vi "Run.vi"(7 "Team Index":i32, 8 "Column":i32, 9 "Row":i32, 10 "View":i32[](array[numeric]) caption="View (Team Index, -1: empty)", 11 "Fortress In":refnum<class "Fortress.lvclass">) -> (0 "Replicated":refnum<class "Square.lvclass">, 1 "Direction":T1, 2 "Action":T2, 3 "Square Out":refnum<class "Square.lvclass">)   [LabVIEW 2015, in "Fortress.lvclass"]
uses:
  Fortress.lvclass
  Square/Square.lvclass
  Type Defs/Action Enum.ctl
  Type Defs/Direction Enum.ctl
  Starter/Starter.lvclass
  Fortress.lvclass/Fortress.ctl
  Common/Common.lvlib
  Type Defs/SB Type Defs.lvlib
panel:
  # "NW\nN\nNE\nE\nSE\nS\nSW\nW"
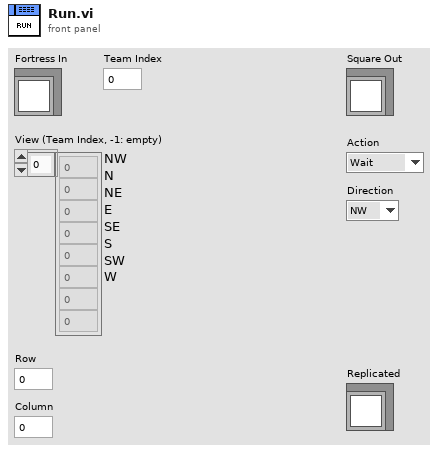
[diagram p1: front panel]
types:
  T1 = typedef "SB Type Defs.lvlib/Direction Enum.ctl" = enum16{"NW", "N", "NE", "E", "SE", "S", "SW", "W"}
  T2 = typedef "SB Type Defs.lvlib/Action Enum.ctl" = enum16{"Wait", "Move", "Attack", "Replicate"}
  T3 = typedef "Common.lvlib/Map DVR.ctl" = refnum<data-value>
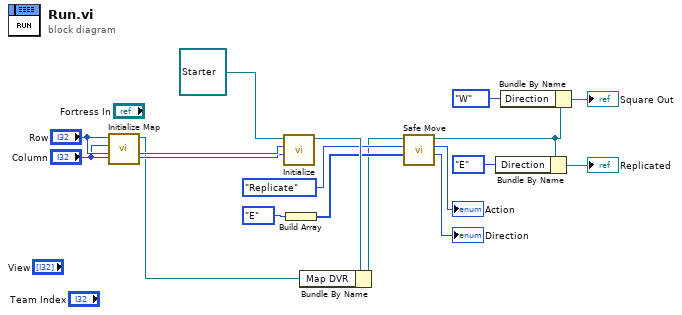
[diagram p0: block diagram]
diagram:
  n1 = call "Initialize Map.vi"("Column"="Column", "Row"="Row") -> ("Map DVR"=w2:T3)  [unwired: 9 in]
  n2 = call-dynamic "Initialize.vi"("Column"="Column", "Row"="Row", "Starter in"=refnum<class "Starter.lvclass"> refnum ("Starter.lvclass")) -> ("Fortress out"=w14:refnum<class "Fortress.lvclass">)  [unwired: 8 in]
  n3 = Build Array(Direction_Enum."E" ("Direction")) -> (w8:T1[])
  n4 = Bundle By Name(cluster=w14, "Map DVR"=w2) -> (w3:refnum<class "Fortress.lvclass">)
  n5 = call "Safe Move.vi"("Directions in"=w8, "Action in"=Action_Enum."Replicate" ("Action"), "Fortress In"=w3) -> ("Direction"=→"Direction":T1, "Action out"=→"Action":T2, "Fortress Out"=w13:refnum<class "Fortress.lvclass">)  [unwired: 5 in, 1 out]
  n6 = Bundle By Name(cluster=w13, "Direction"=Direction_Enum."E") -> (→"Replicated":refnum<class "Fortress.lvclass">)
  n7 = Bundle By Name(cluster=w13, "Direction"=Direction_Enum."W") -> (→"Square Out":refnum<class "Fortress.lvclass">)
